vi "ixon error converter.vi"(4 "Andor error code":u32, 7 "source":string) -> (0 "error out":errorcluster)   [LabVIEW 2016]
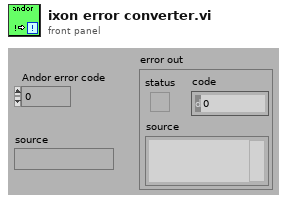
[diagram p1: front panel]
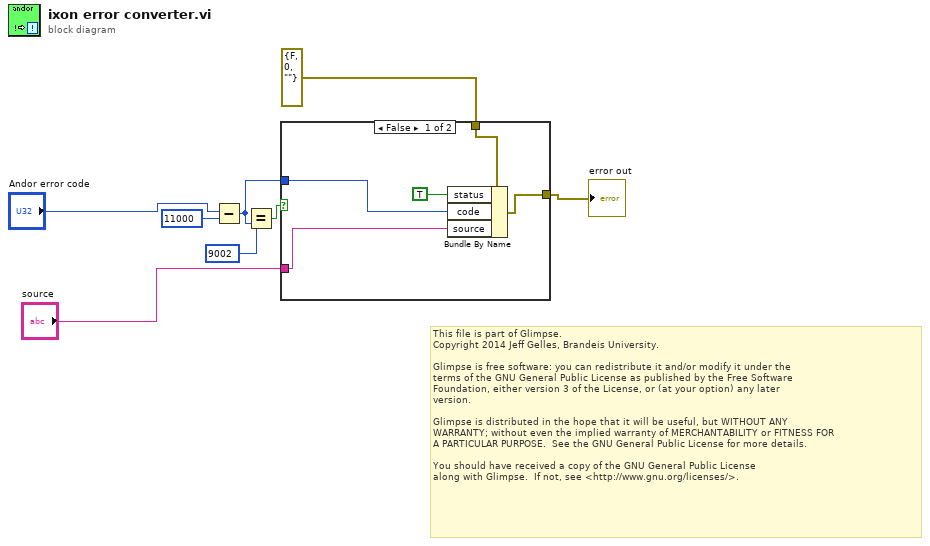
[diagram p0: block diagram]
diagram:
  # "This file is part of Glimpse. \nCopyright 2014 Jeff Gelles, Brandeis University.    \n\nGlimpse is free software: you can redistribute it and/or modify it under the \nterms of the GNU General Public License as published by the Free Software \nFoundation, either version 3 of the License, or (at your option) any later \nversion.\n\nGlimpse is distributed in the hope that it will be useful, but WITHOUT ANY \nWARRANTY; without even the implied warranty of MERCHANTABILITY or FITNESS FOR \nA PARTICULAR PURPOSE.  See the GNU General Public License for more details.\n\nYou should have received a copy of the GNU General Public License\nalong with Glimpse.  If not, see <http://www.gnu.org/licenses/>."
  n1 = Subtract(x="Andor error code", y=u32 11000) -> (x-y=w7:u32)
  n2 = Equal?(x=u32 9002, y=w7) -> (x = y?=w5:bool)
  n3 = case shown="False" w5 {
    tunnel: errorcluster {"status"=FALSE, "code"=0, "source"=""} ("error in (no error) 2") -> [w13 w14]
    tunnel: [w12 w14] -> w1
    tunnel: w7 -> [w10 _]
    tunnel: "source" -> [w9 _]
    frame False {
      n4 = Bundle By Name(cluster=w13, "status"=TRUE, "code"=w10, "source"=w9) -> (w12:errorcluster)
    }
    frame True {
      # "no error"
    }
  }
  "error out" <- w1
